vi "ErrorToString.vi"(2 "error in (no error)":errorcluster) -> (0 "error out":errorcluster, 1 "error string":string)   [LabVIEW 2010]
uses:
  <vilib>/Utility/error.llb/DialogType.ctl
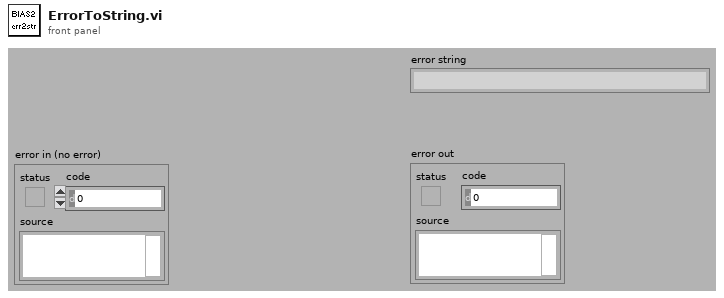
[diagram p1: front panel]
types:
  T1 = typedef "DialogType.ctl" = u16
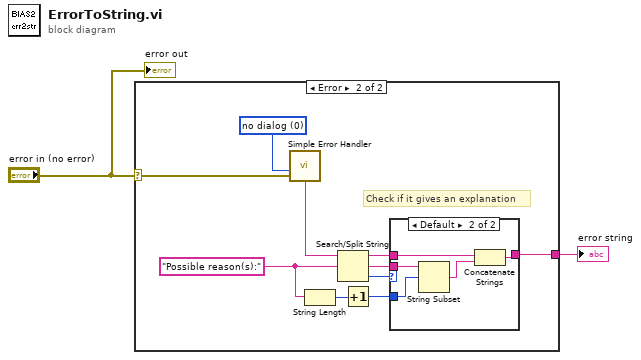
[diagram p0: block diagram]
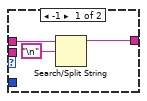
[diagram p3: hidden frame]
diagram:
  n1 = case shown="Error" "error in (no error)" {
    selector: "error in (no error)" -> [_ w3]
    tunnel: [_ w4] -> w2
    frame No Error {
    }
    frame Error {
      w9 = "Possible reason(s):" ("search string/char (-)")
      w12 = T1 0 items=["no dialog", "OK message", "continue or stop message", "OK message + warnings", "continue/stop + warnings"] ("type of dialog (OK msg:1)")
      # "Check if it gives an explanation"
      n2 = call <vilib>:"Simple Error Handler.vi"("type of dialog (OK msg:1)"=w12, "error in (no error)"=w3) -> ("message"=w11:string)  [unwired: 3 in, 4 out]
      n3 = String Length(string=w9) -> (length=w8:i32)
      n4 = Search/Split String(string=w11, search string/char (-)=w9) -> (substring before match=w5:string, match + rest of string=w10:string, offset of match=w6:i32)  [unwired: 1 in]
      n5 = Increment(x=w8) -> (x+1=w7:i32)
      n6 = case shown="Default" w6 {
        tunnel: w10 -> [_ w20]
        tunnel: w7 -> [_ w19]
        tunnel: w5 -> [w15 w17]
        tunnel: [w13 w18] -> w4
        frame -1 {
          n7 = Search/Split String(string=w15, search string/char (-)="\n") -> (substring before match=w13:string)  [unwired: 1 in, 2 out]
        }
        frame Default {
          n8 = String Subset(string=w20, offset (0)=w19) -> (substring=w16:string)  [unwired: 1 in]
          n9 = Concatenate Strings(w17, w16) -> (w18:string)
        }
      }
    }
  }
  "error string" <- w2
  "error out" <- "error in (no error)"
